vi "Configure Modulation (Frequency Shift Keying).vi"(0 "VISA resource name":refnum<visa-resource-name>, 1 "Enable FSK Modulation (T: Enable)":bool=TRUE, 5 "Channel (0: Channel 1)":T1 items=["Channel 1", "Channel 2"], 9 "FSK Modulation Source (0: Internal)":u16(ring) items=["Internal", "External"], 11 "error in (no error)":errorcluster, 12 "Internal Rate (10.00 Hz)":dbl[unit]=10.0 format="%.2f", 13 "Hop Frequency (100.00 Hz)":dbl[unit]=100.0 format="%.2f") -> (4 "VISA resource name out":refnum<visa-resource-name>, 15 "error out":errorcluster)   [LabVIEW 2009, in "Tektronix AFG 3000 Series.lvlib"]
doc: "Configures and enables Frequency-Shift Keying (FSK) modulation. The function generator shifts its output frequency between two present values.\n\n<B> Note:</B>\n\nThe Pulse, Noise, and DC waveform functions are not valid for Configure Modulation (Frequency Shift Keying). \n\n***NOTE: this likely doesn't correctly go back to internal if you set it to external. See \"Configure Modulation (Amplitude).vi\" for how to fix it, if needed."
uses:
  Tektronix AFG 3000 Series.lvlib
  controls.llb/Channel.ctl
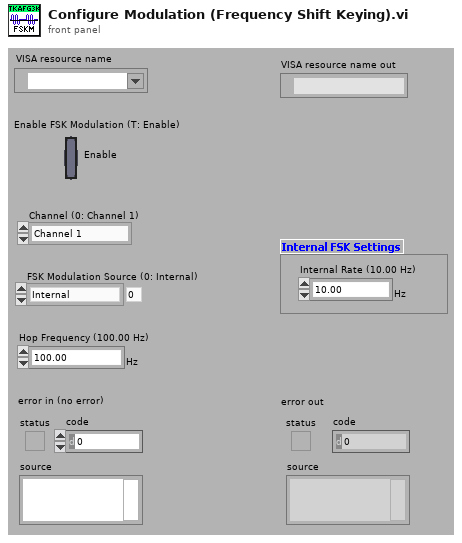
[diagram p1: front panel]
types:
  T1 = typedef "Channel.ctl" = u16
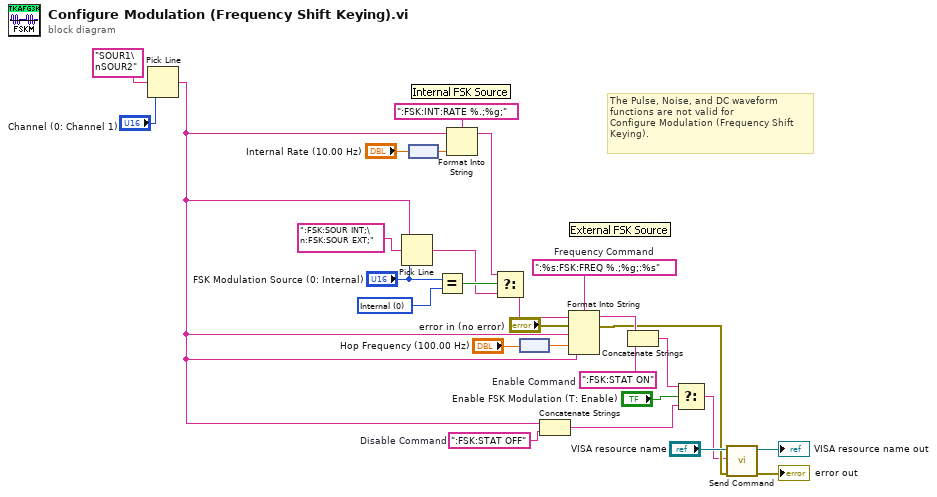
[diagram p0: block diagram]
diagram:
  w24 = ":%s:FSK:FREQ %.;%g;:%s"  # Frequency Command
  w25 = ":FSK:STAT ON"  # Enable Command
  w28 = u16 0 items=["Internal", "External"] ("Source (0: Internal)")
  w13 = ":FSK:STAT OFF"  # Disable Command
  # "The Pulse, Noise, and DC waveform functions are not valid for \nConfigure Modulation (Frequency Shift Keying)."
  n1 = Pick Line(multi-line string="SOUR1\nSOUR2" ("string (\"\")"), line index="Channel (0: Channel 1)") -> (output string=w11:string)  [unwired: 1 out]
  n2 = Pick Line(string ("")=w11, multi-line string=":FSK:SOUR INT;\n:FSK:SOUR EXT;" ("string (\"\")"), line index="FSK Modulation Source (0: Internal)") -> (output string=w16:string)
  n3 = node("Internal Rate (10.00 Hz)") -> (w9:dbl)
  n4 = Equal?(x="FSK Modulation Source (0: Internal)", y=w28) -> (x = y?=w19:bool)
  n5 = Format Into String(format string=":FSK:INT:RATE %.;%g;" ("initial string"), initial string=w11, w9) -> (resulting string=w18:string)  [unwired: 1 in, 1 out]
  n6 = Select(t=w18, s=w19, f=w16) -> (s? t:f=w17:string)
  n7 = node("Hop Frequency (100.00 Hz)") -> (w7:dbl)
  n8 = Concatenate Strings(w11, w13) -> (w12:string)
  n9 = Format Into String(format string=w24, initial string=w17, error in="error in (no error)", w11, w7, w11) -> (resulting string=w26:string, error out=w2:errorcluster)
  n10 = Concatenate Strings(w26, w25) -> (w14:string)
  n11 = Select(t=w14, s="Enable FSK Modulation (T: Enable)", f=w12) -> (s? t:f=w1:string)
  n12 = call "Send Command.vi"("error in (no error)"=w2, "write buffer"=w1, "VISA resource name"="VISA resource name") -> ("error out"=→"error out":errorcluster, "VISA resource name out"=→"VISA resource name out":refnum<visa-resource-name>)  [unwired: 7 out]
